vi "Read Measurement 2 Channels.vi"(8 "error in (no error)":errorcluster, 11 "Osciloscopio in":refnum<class "Osciloscopio.lvclass">) -> (0 "error out":errorcluster, 3 "Osciloscopio out":refnum<class "Osciloscopio.lvclass">)   [LabVIEW 2020, in "Oscilloscope.lvlib" / "Osciloscopio.lvclass"]
uses:
  Osciloscopio.lvclass
  Osciloscopio.lvclass/Osciloscopio.ctl
  <instrlib>/Tektronix TDS 200 1000 2000 Series/Tektronix TDS 200 1000 2000 Series.lvlib
panel:
  out "Measurement":dbl
  out "Units":string
  in  "Channel 1 (1: Channel 1)":i32(ring)=1 items=["Channel 1"=1, "Channel 2"=2, "Channel 3"=3, "Channel 4"=4]
  in  "Channel 2 (2: Channel 2)":i32(ring)=2 items=["Channel 1"=1, "Channel 2"=2, "Channel 3"=3, "Channel 4"=4]
  in  "Measurement Type (0: Phase)":i32(ring) items=["Phase", "Delay", "DelayRR", "DelayRF", "DelayFR", "DelayFF"]
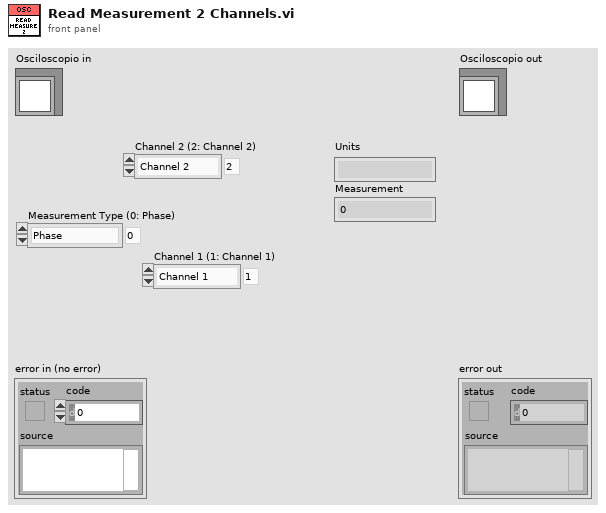
[diagram p1: front panel]
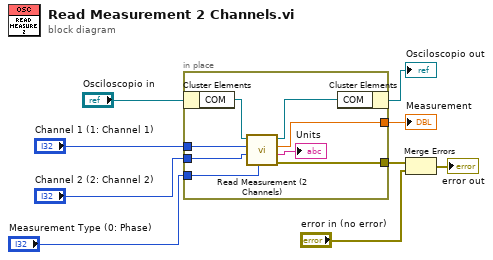
[diagram p0: block diagram]
diagram:
  n1 = in-place {
    in-place-border: [w15] -> w5
    in-place-border: [w13] -> w4
    in-place-border: "Channel 1 (1: Channel 1)" -> [w12]
    in-place-border: "Channel 2 (2: Channel 2)" -> [w11]
    in-place-border: "Measurement Type (0: Phase)" -> [w10]
    n2 = in-place-cluster #1("Osciloscopio in") -> ("COM"=w17:refnum<visa-resource-name>)
    n3 = call <instrlib>:"Read Measurement (2 Channels).vi"("Measurement Type (0: Phase)"=w10, "Channel 2 (2: Channel 2)"=w11, "Channel 1 (1: Channel 1)"=w12, "VISA resource name"=w17) -> ("error out"=w15:errorcluster, "Units"=→"Units":string, "Measurement"=w13:dbl, "VISA resource name out"=w16:refnum<visa-resource-name>)  [unwired: 4 in]
    n4 = in-place-cluster #1("COM"=w16) -> (→"Osciloscopio out":refnum<class "Osciloscopio.lvclass">)
  }
  "Measurement" <- w4
  n5 = Merge Errors(w5, "error in (no error)") -> (→"error out":errorcluster)
